vi "Program.vi"() -> ()   [LabVIEW 2015]
uses:
  Controls/Cluster.ctl
  Controls/States.ctl
panel:
  in  "Knob":u16(knob)=2 scale=0.0..4.0
  in  "Lid":bool
  in  "Drying":bool
  in  "Start":bool
  in  "Stop":bool
  out "Cluster":T1
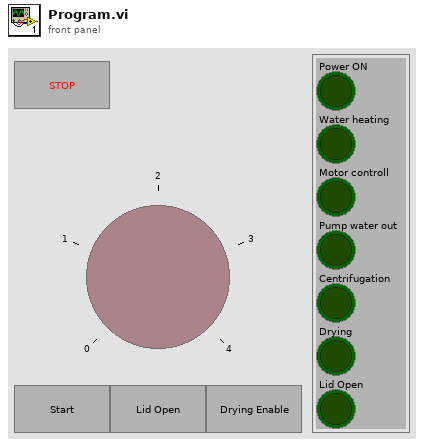
[diagram p1: front panel]
types:
  T1 = typedef "Cluster.ctl" = cluster{"Power ON":bool, "Water heating":bool, "Motor controll":bool, "Pump water out":bool, "Centrifugation":bool, "Drying":bool, "Lid Open":bool}
  T2 = typedef "States.ctl" = enum16{"Init", "Idle", "Cotton", "Silk", "Fast", "Drying"}
  T3 = enum8{"Enabled", "Disabled", "Disabled and Grayed Out"}
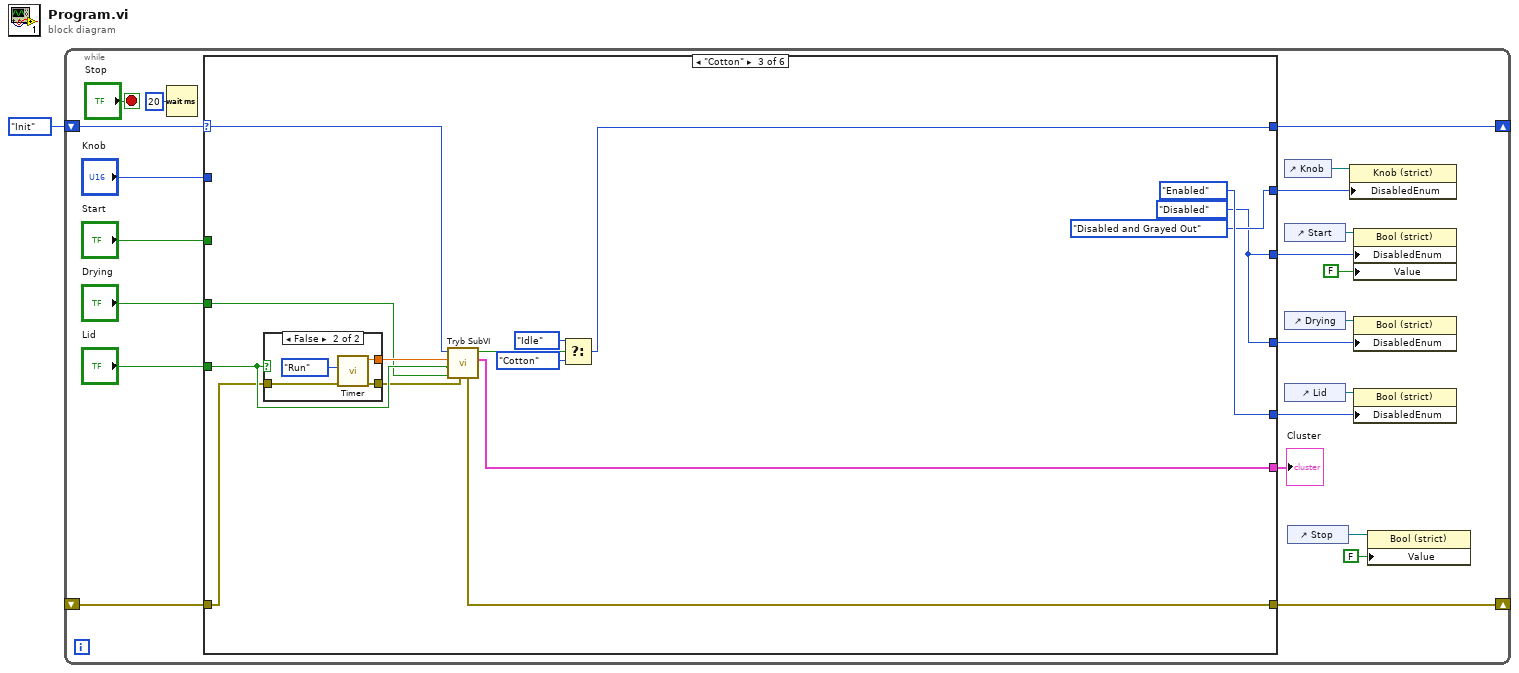
[diagram p0: block diagram]
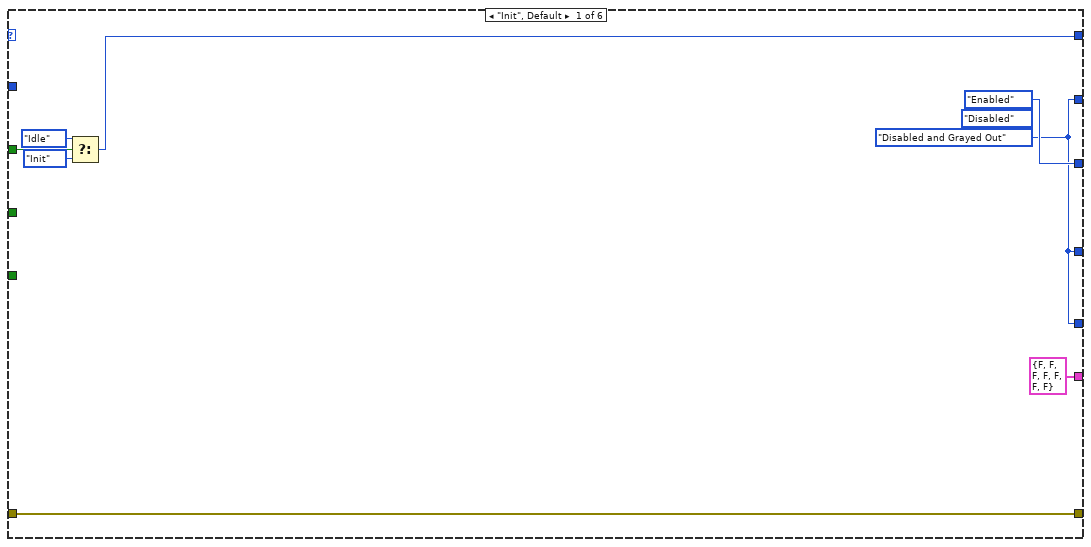
[diagram p2: hidden frame]
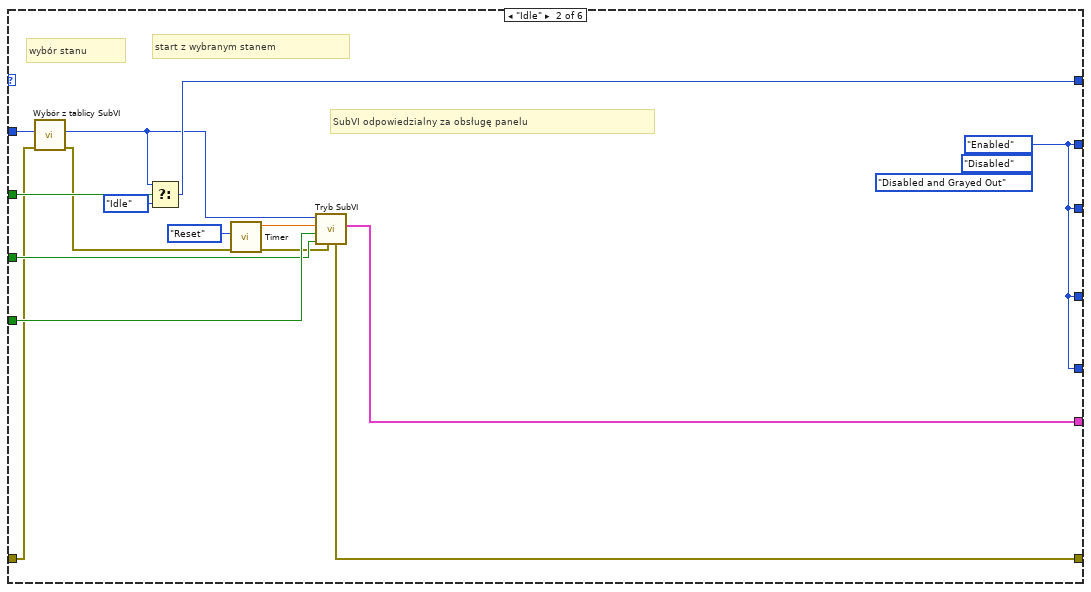
[diagram p3: hidden frame]
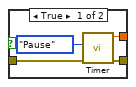
[diagram p4: hidden frame]
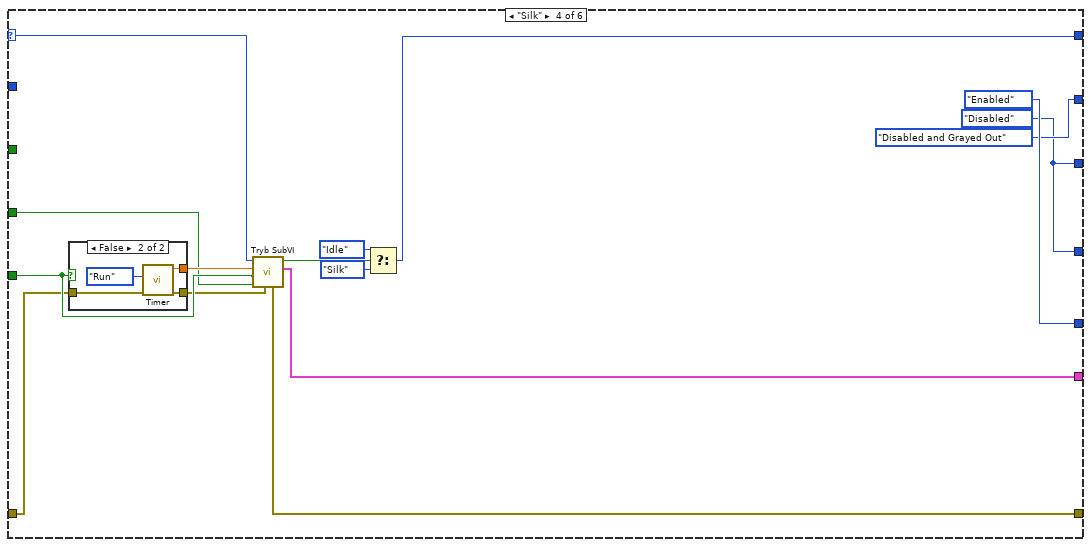
[diagram p5: hidden frame]
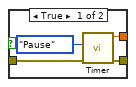
[diagram p6: hidden frame]
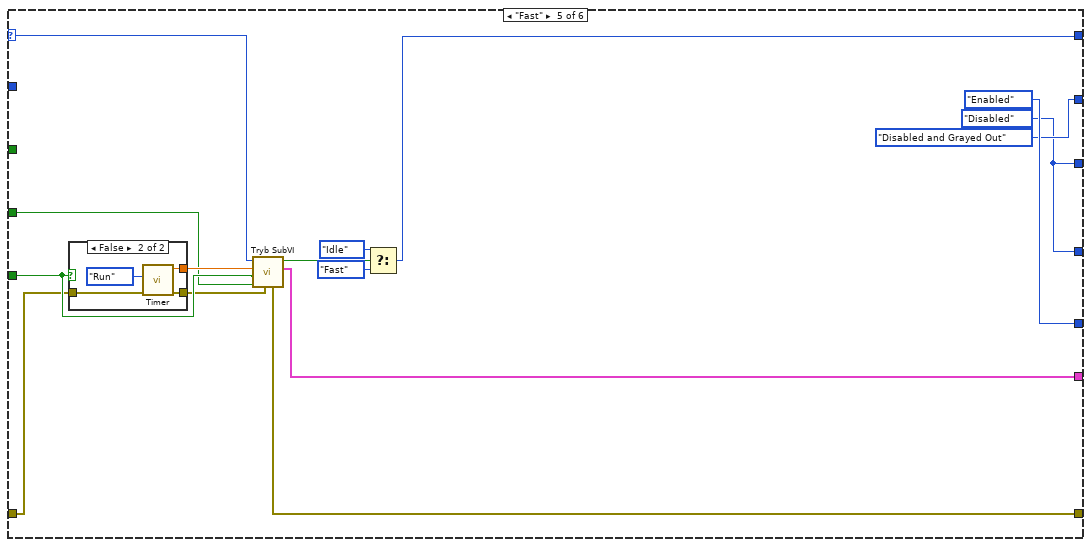
[diagram p7: hidden frame]
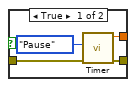
[diagram p8: hidden frame]
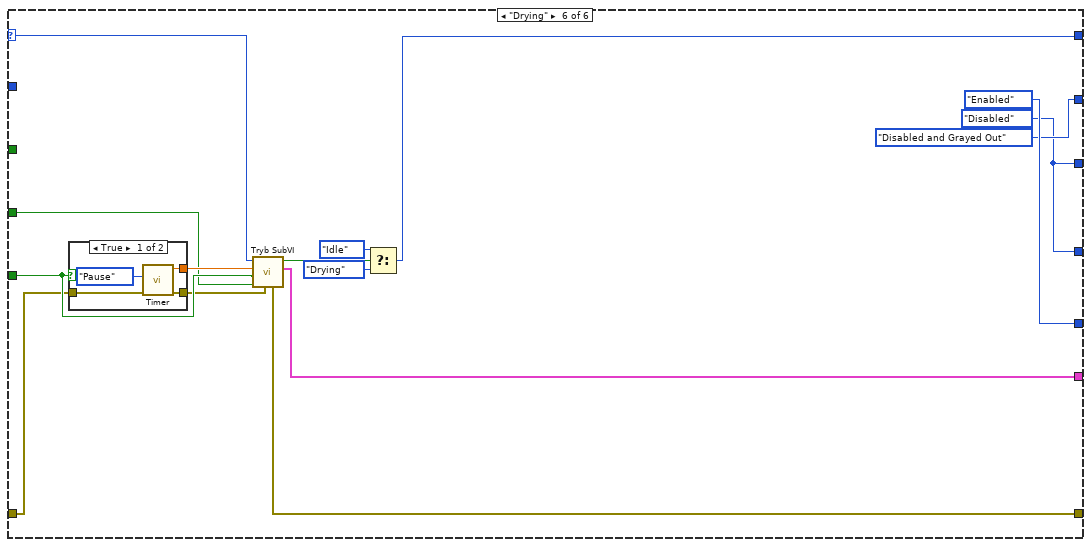
[diagram p9: hidden frame]
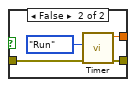
[diagram p10: hidden frame]
diagram:
  n1 = while {
    shift-right: [w16] -> _
    shift-left: States."Init" -> [w21]
    shift-right: [w3] -> _
    shift-left: _ -> [w2]
    stop <- "Stop" stop-if-true
    n2 = Wait (ms)(milliseconds to wait=u32 20) -> ()  [unwired: 1 out]
    n3 = case shown="\"Cotton\"" w21 {
      selector: w21 -> [_ _ w51 w74 w97 w120]
      tunnel: "Knob" -> [_ w42 _ _ _ _]
      tunnel: "Start" -> [w29 w45 _ _ _ _]
      tunnel: "Drying" -> [_ w38 w59 w82 w105 w128]
      tunnel: "Lid" -> [_ w39 w60 w83 w106 w129]
      tunnel: [w28 w41 w53 w76 w99 w122] -> w16
      tunnel: [w25 w44 T3."Disabled and Grayed Out" ("Disabled") T3."Disabled and Grayed Out" ("Disabled") T3."Disabled and Grayed Out" ("Disabled") T3."Disabled and Grayed Out" ("Disabled")] -> w11
      tunnel: [w25 w44 T3."Enabled" ("Disabled") T3."Enabled" ("Disabled") T3."Enabled" ("Disabled") T3."Enabled" ("Disabled")] -> w9
      tunnel: [T3."Enabled" ("Disabled") w44 w52 w75 w98 w121] -> w8
      tunnel: [w25 w44 w52 w75 w98 w121] -> w7
      tunnel: [T1 {"Power ON"=FALSE, "Water heating"=FALSE, "Motor controll"=FALSE, "Pump water out"=FALSE, "Centrifugation"=FALSE, "Drying"=FALSE, "Lid Open"=FALSE} ("Cluster 2") w37 w50 w73 w96 w119] -> w6
      tunnel: [w24 w32 w47 w70 w93 w117] -> w3
      tunnel: w2 -> [w24 w35 w49 w72 w95 w116]
      frame "Init", Default {
        w25 = T3."Disabled and Grayed Out" ("Disabled")
        (unwired) T3."Disabled" ("Disabled")
        n4 = Select(t=States."Idle", s=w29, f=States."Init") -> (s? t:f=w28:T2)
      }
      frame "Idle" {
        (unwired) T3."Disabled and Grayed Out" ("Disabled")
        (unwired) T3."Disabled" ("Disabled")
        w44 = T3."Enabled" ("Disabled")
        # "start z wybranym stanem"
        # "SubVI odpowiedzialny za obsługę panelu"
        # "wybór stanu"
        n5 = call "Wybór z tablicy SubVI.vi"("error in"=w35, "Numeric"=w42) -> ("error out"=w34:errorcluster, "Enum"=w36:T2)  [unwired: 8 in]
        n6 = Select(t=w36, s=w45, f=States."Idle") -> (s? t:f=w41:T2)
        n7 = call "Timer.vi"("error constant"=w34, "Enum"=enum16{"Reset", "Run", "Pause"}."Reset") -> ("error constant 2"=w33:errorcluster, "Stoper"=w40:dbl)  [unwired: 7 in, 1 out]
        n8 = call "Tryb SubVI.vi"("error in"=w33, "Drying"=w38, "Lid"=w39, "Czas"=w40, "Enum"=w36) -> ("output cluster"=w37:T1, "error out"=w32:errorcluster)  [unwired: 4 in, 1 out]
      }
      frame "Cotton" {
        w52 = T3."Disabled" ("Disabled")
        n9 = case shown="False" w60 {
          tunnel: [w64 w68] -> w61
          tunnel: w49 -> [w63 w67]
          tunnel: [w62 w66] -> w48
          frame True {
            n10 = call "Timer.vi"("error constant"=w63, "Enum"=enum16{"Reset", "Run", "Pause"}."Pause") -> ("error constant 2"=w62:errorcluster, "Stoper"=w64:dbl)  [unwired: 7 in, 1 out]
          }
          frame False {
            n11 = call "Timer.vi"("error constant"=w67, "Enum"=enum16{"Reset", "Run", "Pause"}."Run") -> ("error constant 2"=w66:errorcluster, "Stoper"=w68:dbl)  [unwired: 7 in, 1 out]
          }
        }
        n12 = call "Tryb SubVI.vi"("error in"=w48, "Drying"=w59, "Lid"=w60, "Czas"=w61, "Enum"=w51) -> ("output cluster"=w50:T1, "End?"=w54:bool, "error out"=w47:errorcluster)  [unwired: 4 in]
        n13 = Select(t=States."Idle", s=w54, f=States."Cotton") -> (s? t:f=w53:T2)
      }
      frame "Silk" {
        w75 = T3."Disabled" ("Disabled")
        n14 = case shown="False" w83 {
          tunnel: [w87 w91] -> w84
          tunnel: w72 -> [w86 w90]
          tunnel: [w85 w89] -> w71
          frame True {
            n15 = call "Timer.vi"("error constant"=w86, "Enum"=enum16{"Reset", "Run", "Pause"}."Pause") -> ("error constant 2"=w85:errorcluster, "Stoper"=w87:dbl)  [unwired: 7 in, 1 out]
          }
          frame False {
            n16 = call "Timer.vi"("error constant"=w90, "Enum"=enum16{"Reset", "Run", "Pause"}."Run") -> ("error constant 2"=w89:errorcluster, "Stoper"=w91:dbl)  [unwired: 7 in, 1 out]
          }
        }
        n17 = call "Tryb SubVI.vi"("error in"=w71, "Drying"=w82, "Lid"=w83, "Czas"=w84, "Enum"=w74) -> ("output cluster"=w73:T1, "End?"=w77:bool, "error out"=w70:errorcluster)  [unwired: 4 in]
        n18 = Select(t=States."Idle", s=w77, f=States."Silk") -> (s? t:f=w76:T2)
      }
      frame "Fast" {
        w98 = T3."Disabled" ("Disabled")
        n19 = case shown="False" w106 {
          tunnel: [w110 w114] -> w107
          tunnel: w95 -> [w109 w113]
          tunnel: [w108 w112] -> w94
          frame True {
            n20 = call "Timer.vi"("error constant"=w109, "Enum"=enum16{"Reset", "Run", "Pause"}."Pause") -> ("error constant 2"=w108:errorcluster, "Stoper"=w110:dbl)  [unwired: 7 in, 1 out]
          }
          frame False {
            n21 = call "Timer.vi"("error constant"=w113, "Enum"=enum16{"Reset", "Run", "Pause"}."Run") -> ("error constant 2"=w112:errorcluster, "Stoper"=w114:dbl)  [unwired: 7 in, 1 out]
          }
        }
        n22 = call "Tryb SubVI.vi"("error in"=w94, "Drying"=w105, "Lid"=w106, "Czas"=w107, "Enum"=w97) -> ("output cluster"=w96:T1, "End?"=w100:bool, "error out"=w93:errorcluster)  [unwired: 4 in]
        n23 = Select(t=States."Idle", s=w100, f=States."Fast") -> (s? t:f=w99:T2)
      }
      frame "Drying" {
        w121 = T3."Disabled" ("Disabled")
        n24 = case shown="True" w129 {
          tunnel: [w133 w137] -> w130
          tunnel: [w132 w136] -> w118
          tunnel: w116 -> [w131 w135]
          frame True {
            n25 = call "Timer.vi"("error constant"=w131, "Enum"=enum16{"Reset", "Run", "Pause"}."Pause") -> ("error constant 2"=w132:errorcluster, "Stoper"=w133:dbl)  [unwired: 7 in, 1 out]
          }
          frame False {
            n26 = call "Timer.vi"("error constant"=w135, "Enum"=enum16{"Reset", "Run", "Pause"}."Run") -> ("error constant 2"=w136:errorcluster, "Stoper"=w137:dbl)  [unwired: 7 in, 1 out]
          }
        }
        n27 = call "Tryb SubVI.vi"("error in"=w118, "Drying"=w128, "Lid"=w129, "Czas"=w130, "Enum"=w120) -> ("output cluster"=w119:T1, "End?"=w123:bool, "error out"=w117:errorcluster)  [unwired: 4 in]
        n28 = Select(t=States."Idle", s=w123, f=States."Drying") -> (s? t:f=w122:T2)
      }
    }
    "Cluster" <- w6
    n29 = control-ref of="Knob"() -> (w15:refnum<vi>)
    n30 = control-ref of="Start"() -> (w14:refnum<vi>)
    n31 = control-ref of="Drying"() -> (w13:refnum<vi>)
    n32 = control-ref of="Lid"() -> (w12:refnum<vi>)
    n33 = control-ref of="Stop"() -> (w5:refnum<vi>)
    n34 = property class="Knob (strict)"(reference=w15, "DisabledEnum"=w11) -> ()  [unwired: 1 in, 2 out]
    n35 = property class="Bool (strict)"(reference=w14, "DisabledEnum"=w8, "Value"=FALSE) -> ()  [unwired: 1 in, 2 out]
    n36 = property class="Bool (strict)"(reference=w13, "DisabledEnum"=w7) -> ()  [unwired: 1 in, 2 out]
    n37 = property class="Bool (strict)"(reference=w12, "DisabledEnum"=w9) -> ()  [unwired: 1 in, 2 out]
    n38 = property class="Bool (strict)"(reference=w5, "Value"=FALSE) -> ()  [unwired: 1 in, 2 out]
  }
